vi "Template Files Path.vi"() -> (2 "template lib path":path, 3 "xydata ctl path":path)   [LabVIEW 2021, in "MeasurementClient Editor.lvlib"]
uses:
  MeasurementClient Editor.lvlib
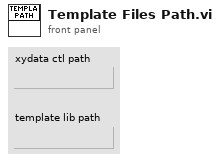
[diagram p1: front panel]
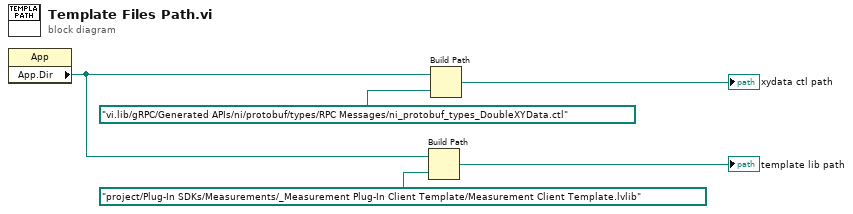
[diagram p0: block diagram]
diagram:
  n1 = property class="App"() -> ("App.Dir"=w1:path)  [unwired: 2 in, 2 out]
  n2 = Build Path(base path=w1, name or relative path=path "project/Plug-In SDKs/Measurements/_Measurement Plug-In Client Template/Measurement Client Template.lvlib") -> (appended path=→"template lib path":path)
  n3 = Build Path(base path=w1, name or relative path=path "vi.lib/gRPC/Generated APIs/ni/protobuf/types/RPC Messages/ni_protobuf_types_DoubleXYData.ctl") -> (appended path=→"xydata ctl path":path)
